vi "case2_selector.vi"(0 "T1":dbl, 2 "T2":dbl, 3 "Delay":dbl) -> (6 "Case 2 selector":enum16{"D=0", "D<T1", "D>=T1"}(ring))   [LabVIEW 2015]
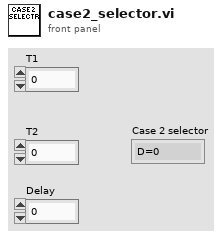
[diagram p1: front panel]
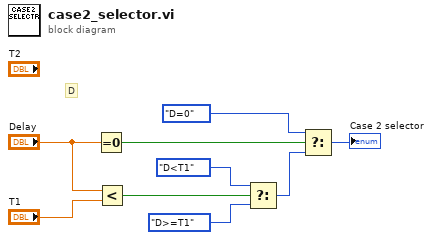
[diagram p0: block diagram]
diagram:
  # "D"
  n1 = Equal To 0?(x="Delay") -> (x = 0?=w7:bool)
  n2 = Less?(x="Delay", y="T1") -> (x < y?=w4:bool)
  n3 = Select(t=enum16{"D=0", "D<T1", "D>=T1"}."D<T1", s=w4, f=enum16{"D=0", "D<T1", "D>=T1"}."D>=T1") -> (s? t:f=w9:enum16{"D=0", "D<T1", "D>=T1"})
  n4 = Select(t=enum16{"D=0", "D<T1", "D>=T1"}."D=0", s=w7, f=w9) -> (s? t:f=→"Case 2 selector":enum16{"D=0", "D<T1", "D>=T1"})
